vi "Get Last.vi"(0 "Executioner in":refnum<class "Executioner.lvclass">, 1 "Linked List Ref":refnum<data-value>, 5 "Active Unique ID":string, 9 "Active Element Index":i32, 11 "error in (no error)":errorcluster) -> (3 "Linked List Ref out":refnum<data-value>, 4 "Executioner out":refnum<class "Executioner.lvclass">, 6 "Active Unique ID out":string, 10 "Active Element Index out":i32, 12 "Restore Point":bool, 13 "Complete":bool, 14 "Stop":bool, 15 "error out":errorcluster)   [LabVIEW 2019, in "Test Executive.lvlib" / "Executioner.lvclass"]
uses:
  <vilib>/gpm_packages/@cs/test-executive/Source/Test Executive/Executioner/Executioner.lvclass
  <vilib>/gpm_packages/@cs/linked-list/Source/Linked List/ILinkedList/ILinked List.lvclass
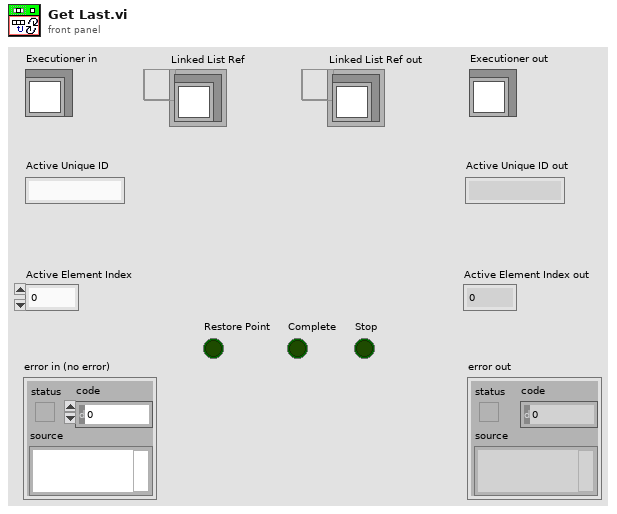
[diagram p1: front panel]
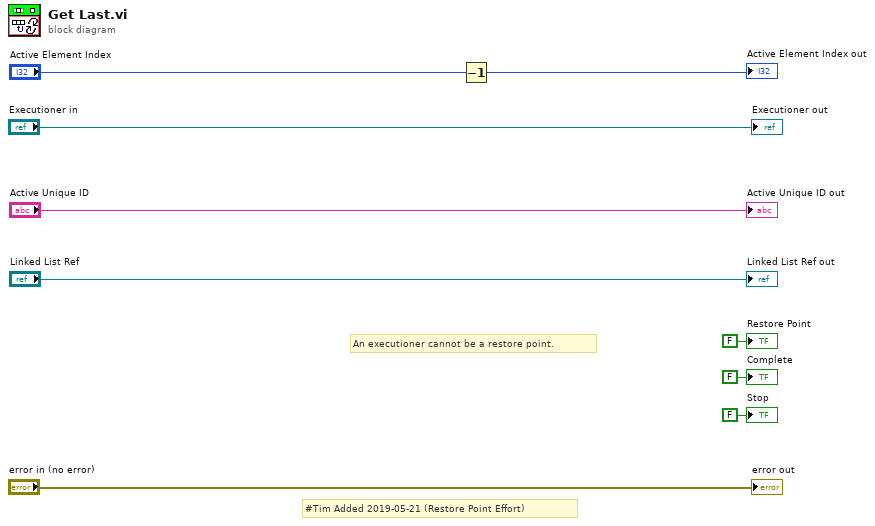
[diagram p0: block diagram]
diagram:
  # "#Tim Added 2019-05-21 (Restore Point Effort)"
  # "An executioner cannot be a restore point."
  n1 = Decrement(x="Active Element Index") -> (x-1=→"Active Element Index out":i32)
  "error out" <- "error in (no error)"
  "Executioner out" <- "Executioner in"
  "Linked List Ref out" <- "Linked List Ref"
  "Active Unique ID out" <- "Active Unique ID"
  "Restore Point" <- FALSE ("Found")
  "Complete" <- FALSE ("Complete")
  "Stop" <- FALSE ("Stop")
